vi "OpenCloseSymbols.vi"(8 "error in (no error)":errorcluster, 11 "Tree ref":refnum<vi>) -> (0 "error out":errorcluster, 3 "Tree ref out":refnum<vi>)   [LabVIEW 2020, in "ScriptManager.lvlib"]
uses:
  ScriptManager.lvlib
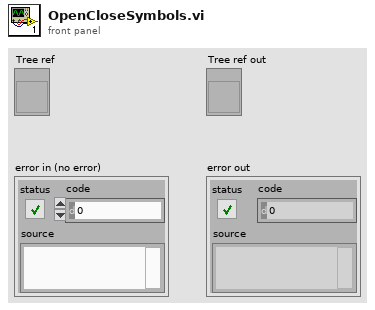
[diagram p1: front panel]
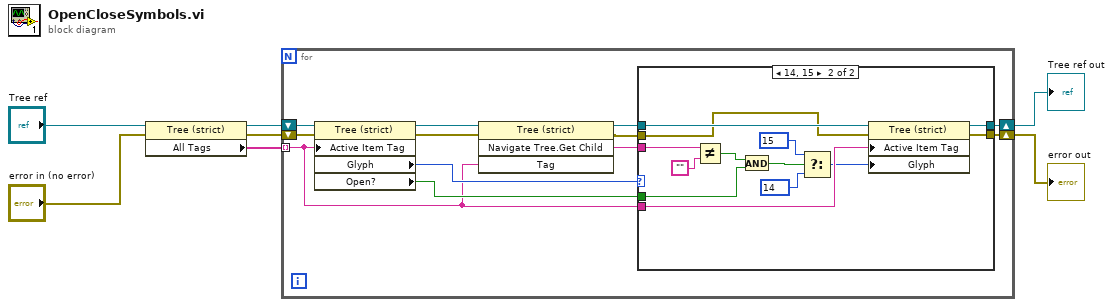
[diagram p0: block diagram]
diagram:
  n1 = property class="Tree (strict)"(reference="Tree ref", error in="error in (no error)") -> (reference out=w5:refnum<vi>, error out=w4:errorcluster, "All Tags"=w6:string[])
  n2 = for {
    tunnel: w6 -> [w11] mode=indexing
    shift-right: [w9] -> w1
    shift-left: w4 -> [w17]
    shift-right: [w8] -> w2
    shift-left: w5 -> [w19]
    n3 = property class="Tree (strict)"(reference=w19, error in=w17, "Active Item Tag"=w11) -> (reference out=w18:refnum<vi>, error out=w16:errorcluster, "Glyph"=w15:i32, "Open?"=w13:bool)
    n4 = invoke class="Tree (strict)" method="Navigate Tree.Get Child"(reference=w18, error in=w16, "Tag"=w11) -> (reference out=w12:refnum<vi>, error out=w10:errorcluster, "Navigate Tree:Get Child"=w14:string)  [unwired: 1 in, 1 out]
    n5 = case shown="14, 15" w15 {
      tunnel: w14 -> [_ w26]
      tunnel: w13 -> [_ w33]
      tunnel: w12 -> [w21 w29]
      tunnel: w11 -> [_ w28]
      tunnel: w10 -> [w20 w24]
      tunnel: [w20 w23] -> w9
      tunnel: [w21 w22] -> w8
      frame Default {
      }
      frame 14, 15 {
        n6 = Not Equal?(x=w26, y="") -> (x != y?=w34:bool)
        n7 = And(x=w34, y=w33) -> (x .and. y?=w32:bool)
        n8 = Select(t=15, s=w32, f=14) -> (s? t:f=w27:i32)
        n9 = property class="Tree (strict)"(reference=w29, error in=w24, "Active Item Tag"=w28, "Glyph"=w27) -> (reference out=w22:refnum<vi>, error out=w23:errorcluster)
      }
    }
  }
  "Tree ref out" <- w2
  "error out" <- w1
